vi "ndipolaris Stop Tracking.vi"(8 "error in (no error)":errorcluster, 11 "VISA resource name":refnum<visa-resource-name>) -> (0 "error out":errorcluster, 3 "VISA resource out":refnum<visa-resource-name>)   [LabVIEW 2013]
doc: "This VI will stop the acquisition of transformations and the instrument will leave the tracking state. After this VI has executed the instrument will be in the setup state."
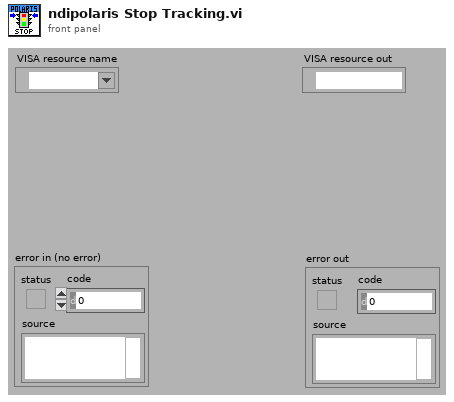
[diagram p1: front panel]
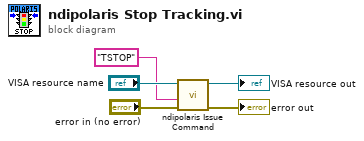
[diagram p0: block diagram]
diagram:
  n1 = call <instrlib>:"ndipolaris Issue Command.vi"("error in (no error)"="error in (no error)", "Write Buffer"="TSTOP" ("string"), "VISA resource name"="VISA resource name") -> ("error out"=→"error out":errorcluster, "VISA resource out"=→"VISA resource out":refnum<visa-resource-name>)  [unwired: 6 in, 1 out]
